vi "Project XML Editor.vi"() -> ()   [LabVIEW 2019, in "Project XML Editor.lvclass"]
uses:
  Project XML Editor.lvclass
  TypeDefs/Dependency Parameters.ctl
  <vilib>/xml/NI_XML.lvlib
  <resource>/objmgr/DOMUserDefRef.rc
  <vilib>/xml/Close Reference(NNMap).vi
panel:
  out "error out":errorcluster
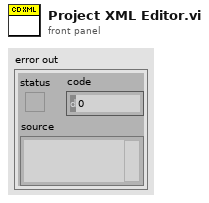
[diagram p1: front panel]
types:
  T1 = typedef "Project XML Editor.lvclass/Dependency Parameters.ctl" = cluster{"Supported Target":string, "RT System Destination":string, "Source Path (Relative)":string}
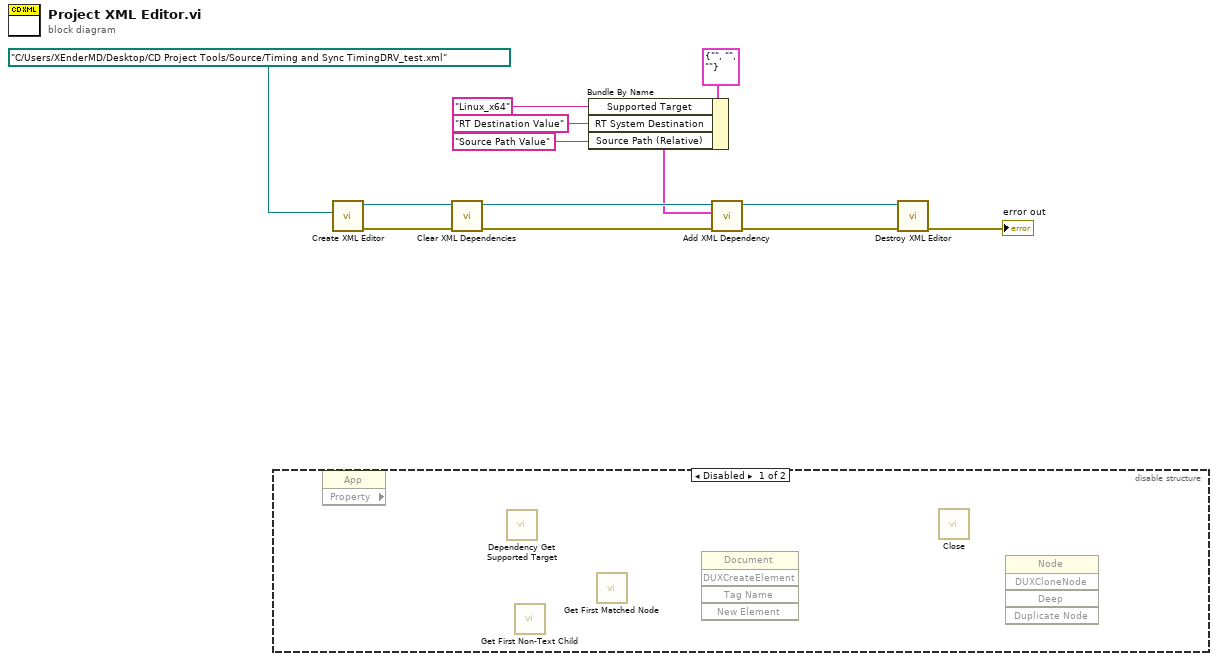
[diagram p0: block diagram]
diagram:
  n1 = disable-structure shown="Disabled" {
    frame Disabled {
      n2 = property class="App" props=[]() -> ()  [unwired: 2 in, 3 out]
      n3 = call "Dependency Get Supported Target.vi"() -> ()  [unwired: 9 in, 3 out]
      n4 = call <vilib>:"Get First Non-Text Child.vi"() -> ()  [unwired: 8 in, 4 out]
      n5 = call <vilib>:"Get First Matched Node.vi"() -> ()  [unwired: 9 in, 3 out]
      n6 = invoke class="Document" method="DUXCreateElement"() -> ()  [unwired: 5 in, 5 out]
      n7 = call-poly <vilib>:"Close.vi"() -> ()  [unwired: 9 in, 1 out]
      n8 = invoke class="Node" method="DUXCloneNode"() -> ()  [unwired: 5 in, 5 out]
    }
    frame Enabled {
    }
  }
  n9 = call "Create XML Editor.vi"("XML Path"=path "C:/Users/XEnderMD/Desktop/CD Project Tools/Source/Timing and Sync TimingDRV_test.xml") -> ("error out"=w8:errorcluster, "Project XML Editor out"=w9:refnum<class "Project XML Editor.lvclass">)  [unwired: 9 in]
  n10 = call "Clear XML Dependencies.vi"("error in (no error)"=w8, "Project XML Editor in"=w9) -> ("error out"=w6:errorcluster, "Project XML Editor out"=w7:refnum<class "Project XML Editor.lvclass">)  [unwired: 8 in]
  n11 = Bundle By Name(cluster=T1 {"Supported Target"="", "RT System Destination"="", "Source Path (Relative)"=""} ("Dependency Parameters"), "Supported Target"="Linux_x64", "RT System Destination"="RT Destination Value", "Source Path (Relative)"="Source Path Value") -> (w1:T1)
  n12 = call "Add XML Dependency.vi"("error in (no error)"=w6, "Dependency Parameters"=w1, "Project XML Editor in"=w7) -> ("error out"=w10:errorcluster, "Project XML Editor out"=w11:refnum<class "Project XML Editor.lvclass">)  [unwired: 7 in]
  n13 = call "Destroy XML Editor.vi"("error in (no error)"=w10, "Project XML Editor in"=w11) -> ("error out"=→"error out":errorcluster)  [unwired: 9 in]
